vi "Test Initialize Rings.vi"(8 "error in":errorcluster) -> (0 "error out":errorcluster)   [LabVIEW 2020]
uses:
  <vilib>/addons/_JKI Toolkits/Caraya/classes/Test/Test.lvclass
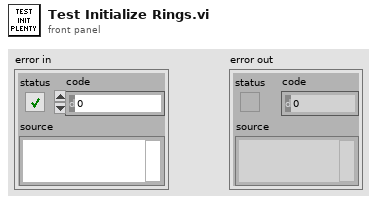
[diagram p1: front panel]
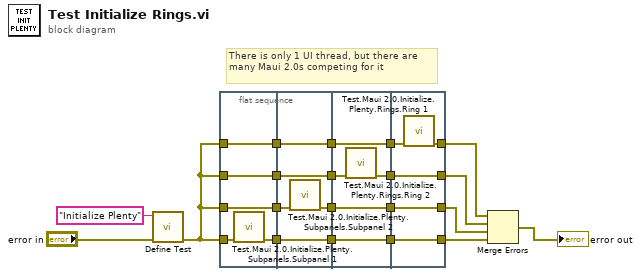
[diagram p0: block diagram]
diagram:
  # "There is only 1 UI thread, but there are many Maui 2.0s competing for it"
  n1 = call <vilib>:"Define Test.vi"("error in (no error)"="error in", "Label (VI Title)"="Initialize Plenty") -> ("error out"=w2:errorcluster)  [unwired: 9 in]
  n2 = flat-sequence {
    tunnel: w2 -> [w25]
    tunnel: w2 -> [w24]
    tunnel: [w24] -> w18
    tunnel: w2 -> [w23]
    tunnel: [w23] -> w17
    tunnel: w2 -> [w22]
    tunnel: [w22] -> w15
    tunnel: [w21] -> w7
    tunnel: w18 -> [w30]
    tunnel: w17 -> [w29]
    tunnel: [w29] -> w16
    tunnel: w15 -> [w28]
    tunnel: [w28] -> w14
    tunnel: [w27] -> w10
    tunnel: [w26] -> w8
    tunnel: w7 -> [w26]
    tunnel: w16 -> [w35]
    tunnel: w14 -> [w34]
    tunnel: [w34] -> w13
    tunnel: [w33] -> w12
    tunnel: [w32] -> w11
    tunnel: w10 -> [w32]
    tunnel: [w31] -> w9
    tunnel: w8 -> [w31]
    tunnel: w13 -> [w40]
    tunnel: [w39] -> w3
    tunnel: [w38] -> w4
    tunnel: w12 -> [w38]
    tunnel: [w37] -> w5
    tunnel: w11 -> [w37]
    tunnel: [w36] -> w6
    tunnel: w9 -> [w36]
    frame #0 {
      n3 = call "Test.Maui 2.0.Initialize.Plenty.Subpanels.Subpanel 1.vi"("error in"=w25) -> ("error out"=w21:errorcluster)  [unwired: 10 in]
    }
    frame #1 {
      n4 = call "Test.Maui 2.0.Initialize.Plenty.Subpanels.Subpanel 2.vi"("error in"=w30) -> ("error out"=w27:errorcluster)  [unwired: 10 in]
    }
    frame #2 {
      n5 = call "Test.Maui 2.0.Initialize.Plenty.Rings.Ring 2.vi"("error in"=w35) -> ("error out"=w33:errorcluster)  [unwired: 10 in]
    }
    frame #3 {
      n6 = call "Test.Maui 2.0.Initialize.Plenty.Rings.Ring 1.vi"("error in"=w40) -> ("error out"=w39:errorcluster)  [unwired: 10 in]
    }
  }
  n7 = Merge Errors(w3, w4, w5, w6) -> (→"error out":errorcluster)
